vi "From CSV File.vi"(8 "error in (no error)":errorcluster, 9 "Path":path, 10 "engine in":refnum<class "engine configuration.lvclass">, 11 "tag select module editor node in":refnum<class "tag select module editor node.lvclass">) -> (0 "error out":errorcluster, 1 "Update":bool, 2 "engine out":refnum<class "engine configuration.lvclass">, 3 "tag select module editor node out":refnum<class "tag select module editor node.lvclass">)   [LabVIEW 2015, in "tag select module editor node.lvclass"]
uses:
  tag select module editor node.lvclass
  <vilib>/NI/Module Execution Interface/Engine Configuration/engine configuration.lvclass
  module/configuration/tag select module configuration.lvclass
  <vilib>/NI/Configuration Framework/serializable configuration/NISE_CEF_serializable configuration.lvclass/NISE_CEF_serializable configuration.ctl
  module/configuration/tag select module configuration.lvclass/tag select module configuration.ctl
  module/configuration/Read tag select.vi
  <vilib>/Utility/LVClass/Get LV Class Name.vi
  <vilib>/NI/Configuration Framework/error generator/NISE_error generator.vi
  <vilib>/NI/Tag Bus Module Framework/channel/TBM channel.lvclass
  <vilib>/NI/Configuration Framework/serializable configuration/NISE_CEF_serializable configuration.lvclass
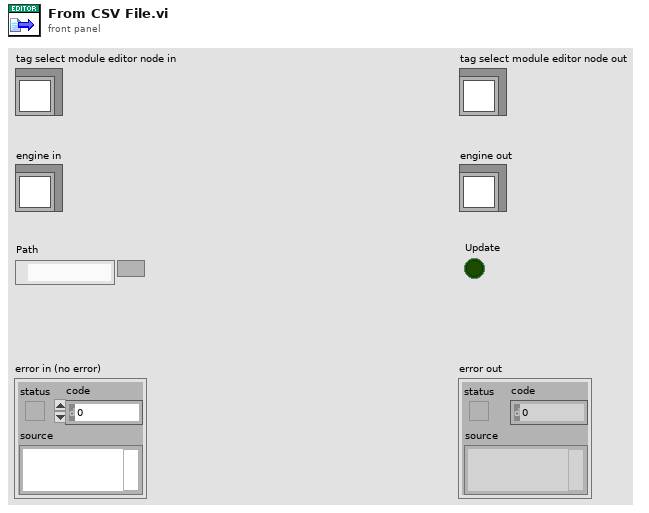
[diagram p1: front panel]
types:
  T1 = typedef "tag select module configuration.lvclass/tag select configuration.ctl" = cluster{"tag select name":string, "data type":T2, "output":refnum<class "TBM channel.lvclass">, "select":refnum<class "TBM channel.lvclass">, "input channels":refnum<class "TBM channel.lvclass">[]}
  T2 = typedef "tag bus.lvlib/tag descriptor.lvclass/Data Type.ctl" = enum16{"Double", "Single", "I64", "I32", "I16", "I8", "U64", "U32", "U16", "U8", "Boolean", "String", "Array of Double", "Array of Single", "Array of I64", "Array of I32", "Array of I16", "Array of I8", "Array of U64", "Array of U32", "Array of U16", "Array of U8", "Array of Boolean", "Array of String"}
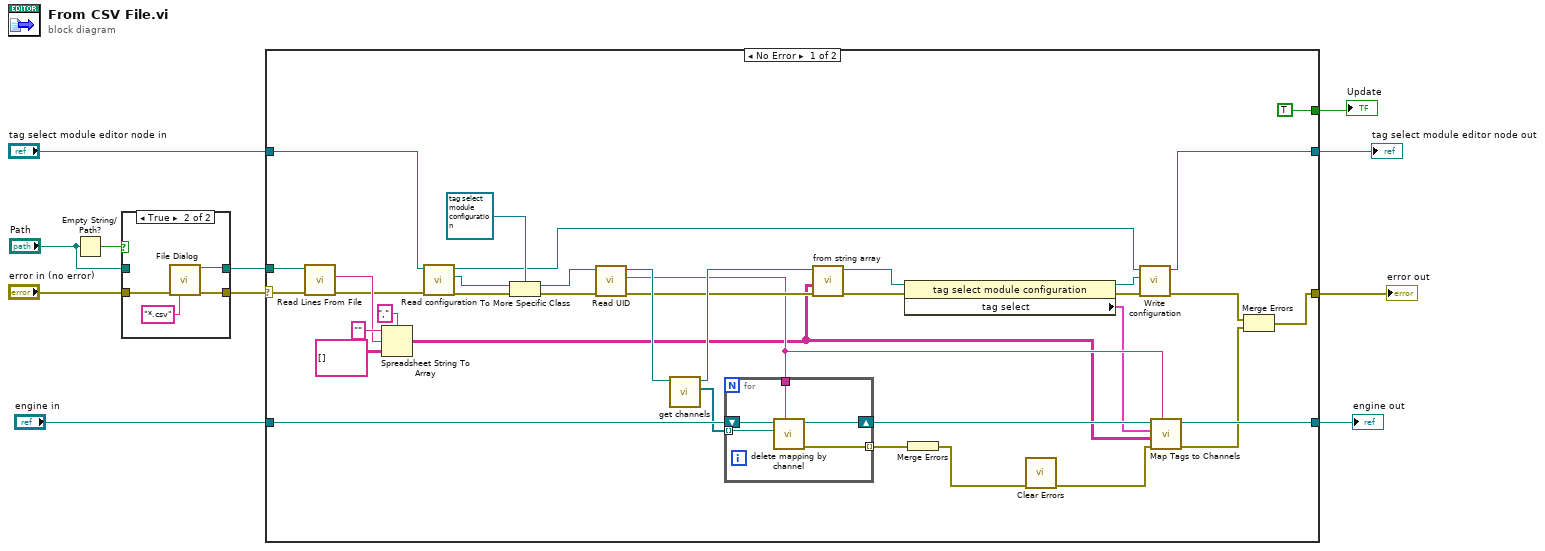
[diagram p0: block diagram]
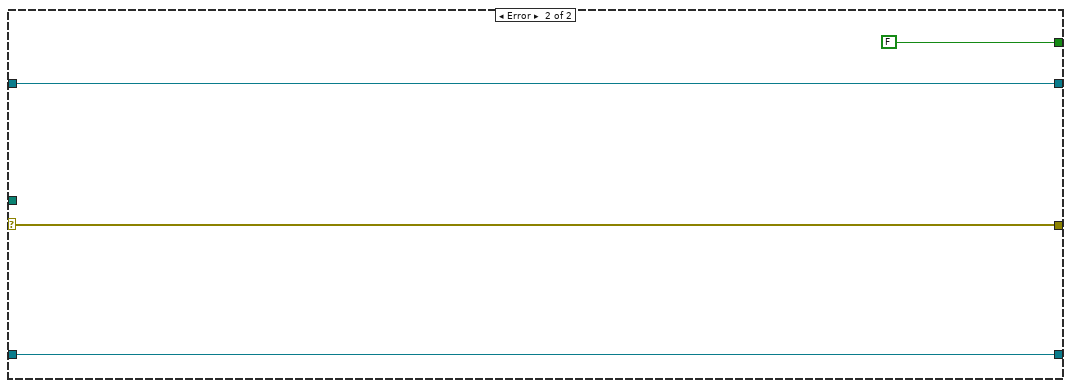
[diagram p2: hidden frame]
diagram:
  n1 = Empty String/Path?(string/path="Path") -> (empty?=w11:bool)
  n2 = case shown="True" w11 {
    tunnel: "error in (no error)" -> [w12 w16]
    tunnel: [w12 w15] -> w7
    tunnel: [w13 w14] -> w5
    tunnel: "Path" -> [w13 _]
    frame False {
    }
    frame True {
      n3 = call "File Dialog"("error in"=w16, "pattern (all files)"="*.csv") -> ("selected path"=w14:path, "error out"=w15:errorcluster)  [unwired: 10 in, 2 out]
    }
  }
  n4 = case shown="No Error" w7 {
    selector: w7 -> [w53 w59]
    tunnel: "tag select module editor node in" -> [w48 w60]
    tunnel: "engine in" -> [w40 w61]
    tunnel: w5 -> [w52 _]
    tunnel: [TRUE FALSE] -> w4
    tunnel: [w28 w61] -> w3
    tunnel: [w32 w60] -> w2
    tunnel: [w26 w59] -> w1
    frame No Error {
      n5 = call <vilib>:"Read Lines From File.vi"("file path (dialog if empty)"=w52, "error in (not an error)"=w53) -> ("line string"=w49:string, "error out"=w47:errorcluster)  [unwired: 5 in, 1 out]
      n6 = Spreadsheet String To Array(delimiter (Tab)=",", format string="", spreadsheet string=w49, array type (2D Dbl)=string[][] [] ("type (empty)")) -> (array=w19:string[][])
      n7 = call-dynamic "Read configuration.vi"("error in"=w47, "tag select module editor node in"=w48) -> ("error out"=w46:errorcluster, "configuration"=w45:refnum<class "NISE_CEF_serializable configuration.lvclass">, "tag select module editor node out"=w33:refnum<class "tag select module editor node.lvclass">)  [unwired: 7 in]
      n8 = To More Specific Class(target class=refnum<class "tag select module configuration.lvclass"> refnum ("tag select module configuration"), reference=w45, error in=w46) -> (specific class reference=w42:refnum<class "tag select module configuration.lvclass">, error out=w43:errorcluster)
      n9 = call <vilib>:"Read UID.vi"("error in"=w43, "configuration in"=w42) -> ("error out"=w35:errorcluster, "instance id"=w30:string, "configuration out"=w41:refnum<class "tag select module configuration.lvclass">)  [unwired: 7 in]
      n10 = call-dynamic "get channels.vi"("tag select module configuration in"=w41) -> ("channels"=w39:refnum<class "TBM channel.lvclass">[], "tag select module configuration out"=w36:refnum<class "tag select module configuration.lvclass">)  [unwired: 9 in]
      n11 = for {
        shift-right: [w57] -> w29
        shift-left: w40 -> [w58]
        tunnel: w30 -> [w56]
        tunnel: w39 -> [w55] mode=indexing
        tunnel: [w54] -> w38 mode=indexing
        n12 = call <vilib>:"delete mapping by channel.vi"("owner ID"=w56, "channel"=w55, "engine configuration in"=w58) -> ("error out"=w54:errorcluster, "engine configuration out"=w57:refnum<class "engine configuration.lvclass">)  [unwired: 7 in]
      }
      n13 = call-dynamic "from string array.vi"("error in (no error)"=w35, "String Array"=w19, "module configuration in"=w36) -> ("error out"=w23:errorcluster, "module configuration out"=w24:refnum<class "tag select module configuration.lvclass">)  [unwired: 7 in]
      n14 = property class="tag select module configuration"(reference=w24, error in=w23) -> (reference out=w21:refnum<class "tag select module configuration.lvclass">, error out=w22:errorcluster, "tag select"=w20:T1[])
      n15 = Merge Errors(w38) -> (w37:errorcluster)
      n16 = call <vilib>:"Clear Errors.vi"("error in (no error)"=w37) -> ("error out"=w18:errorcluster)  [unwired: 5 in, 1 out]
      n17 = call-dynamic "Write configuration.vi"("error in"=w22, "configuration"=w21, "tag select module editor node in"=w33) -> ("error out"=w27:errorcluster, "tag select module editor node out"=w32:refnum<class "tag select module editor node.lvclass">)  [unwired: 7 in]
      n18 = call "Map Tags to Channels.vi"("instance id"=w30, "error in (no error)"=w18, "String Array"=w19, "tag select"=w20, "engine in"=w29) -> ("error out"=w25:errorcluster, "engine out"=w28:refnum<class "engine configuration.lvclass">)  [unwired: 5 in]
      n19 = Merge Errors(w27, w25) -> (w26:errorcluster)
    }
    frame Error {
    }
  }
  "error out" <- w1
  "tag select module editor node out" <- w2
  "Update" <- w4
  "engine out" <- w3
